vi "Lower_Stop.vi"(10 "Motion in":refnum<class "Motion.lvclass">, 11 "I-O in":refnum<class "I-O.lvclass">) -> (2 "Motion out":refnum<class "Motion.lvclass">, 3 "I-O out":refnum<class "I-O.lvclass">)   [LabVIEW 2016]
uses:
  Classes/Controllers/I-O/Copy of I-O Folder/I-O.lvclass
  Classes/Controllers/Motion/Copy of Motion Folder/Motion.lvclass
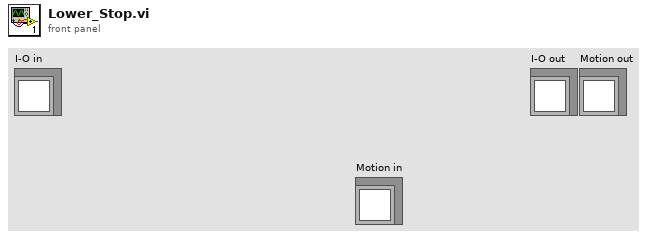
[diagram p1: front panel]
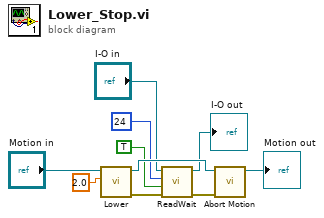
[diagram p0: block diagram]
diagram:
  n1 = call-dynamic "Lower.vi"("Speed"=2.0, "Motion in"="Motion in") -> ("error out"=w9:errorcluster, "Motion out"=w8:refnum<class "Motion.lvclass">)  [unwired: 8 in]
  n2 = call "ReadWait.vi"("error in (no error)"=w9, "Value"=TRUE, "Read"=24, "I-O in"="I-O in") -> ("error out"=w10:errorcluster, "I-O out"=→"I-O out":refnum<class "I-O.lvclass">)  [unwired: 6 in]
  n3 = call-dynamic "Abort Motion.vi"("error in (no error)"=w10, "Motion in"=w8) -> ("Motion out"=→"Motion out":refnum<class "Motion.lvclass">)  [unwired: 8 in, 1 out]
